vi "Write Local Search .vi"(8 "error in (no error)":errorcluster, 10 "Local Search":T1, 11 "GA in":refnum<class "GA.lvclass">) -> (0 "error out":errorcluster, 3 "GA out":refnum<class "GA.lvclass">)   [LabVIEW 2013, in "GA.lvclass"]
uses:
  GA.lvclass
  GA/Controls/Local Search Type.ctl
  GA.lvclass/GA.ctl
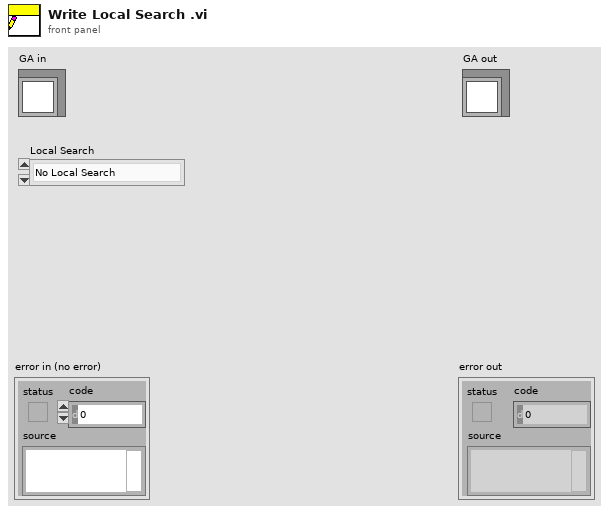
[diagram p1: front panel]
types:
  T1 = typedef "Local Search Type.ctl" = enum16{"No Local Search", "SA Population", "IRH3T(Pop)", "IRH3T(Best Solution)", "SA Best Solution", "SA Random Solution", "SA Random 3 Solutions", "SA Hybrid"}
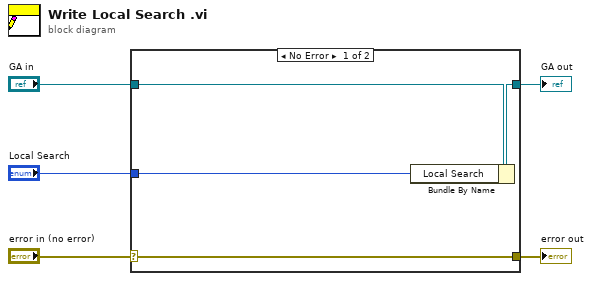
[diagram p0: block diagram]
diagram:
  n1 = case shown="No Error" "error in (no error)" {
    selector: "error in (no error)" -> [w9 w10]
    tunnel: [w9 w10] -> w4
    tunnel: [w7 w11] -> w2
    tunnel: "GA in" -> [w8 w11]
    tunnel: "Local Search" -> [w6 _]
    frame No Error {
      n2 = Bundle By Name(cluster=w8, "Local Search"=w6) -> (w7:refnum<class "GA.lvclass">)
    }
    frame Error {
    }
  }
  "error out" <- w4
  "GA out" <- w2
